vi "Known Hosts.vi"(8 "Error In":errorcluster, 11 "Session In":refnum<class "Session.lvclass">) -> (0 "Error Out":errorcluster, 2 "Known Hosts":refnum<class "KnownHosts.lvclass">, 3 "Session Out":refnum<class "Session.lvclass">)   [LabVIEW 2017, in "LabSSH2.lvlib" / "Session.lvclass"]
uses:
  Session.lvclass
  KnownHosts/KnownHosts.lvclass
  Session.lvclass/Session.ctl
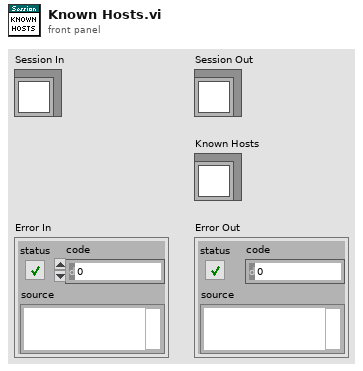
[diagram p1: front panel]
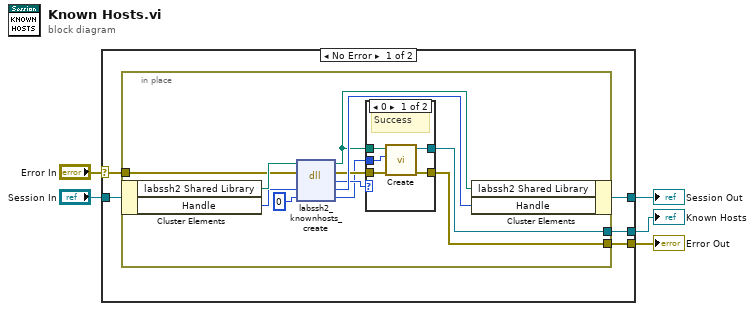
[diagram p0: block diagram]
diagram:
  n1 = case shown="No Error" "Error In" {
    selector: "Error In" -> [w9 w28]
    tunnel: "Session In" -> [w10 w29]
    tunnel: [w6 w29] -> w3
    tunnel: [w8 w28] -> w2
    tunnel: [w7 _] -> w1
    frame No Error {
      n2 = in-place {
        in-place-border: w9 -> [w19]
        in-place-border: [w13] -> w8
        in-place-border: [w12] -> w7
        n3 = in-place-cluster #1(w10) -> ("labssh2 Shared Library"=w20:path, "Handle"=w18:u64)
        n4 = dll-call lib="D:/Users/cfield/Code/Field R&D Services/SSH/LabSSH2/LabVIEW/trunk/src/LabSSH2/Private/labssh2.*" fn="labssh2_knownhosts_create"(path in=w20, error in=w19, "session"=w18, "handle"=u64 0) -> (path out=w11:path, error out=w15:errorcluster, "status"=w16:i32, "session"=w17:u64, "handle"=w14:u64)  [unwired: 1 in]
        n5 = case shown="0" w16 {
          tunnel: w15 -> [w26 w27]
          tunnel: [w24 w27] -> w13
          tunnel: w14 -> [w23 _]
          tunnel: [w25 _] -> w12
          tunnel: w11 -> [w22 _]
          frame 0 {
            # "Success"
            n6 = call "Create.vi"("Error In"=w26, "Handle"=w23, "labssh2 Shared Library"=w22) -> ("Error Out"=w24:errorcluster, "Known Hosts"=w25:refnum<class "KnownHosts.lvclass">)  [unwired: 7 in]
          }
          frame -1, Default {
            # "Error"
          }
        }
        n7 = in-place-cluster #1("labssh2 Shared Library"=w11, "Handle"=w17) -> (w6:refnum<class "Session.lvclass">)
      }
    }
    frame Error {
    }
  }
  "Error Out" <- w2
  "Known Hosts" <- w1
  "Session Out" <- w3
